vi "Autonomous Independent.vi"() -> ()   [LabVIEW 2017]
doc: "This VI is called when autonomous begins, and will automatically be terminated when autonomous ends. You can carry out timed or sensor driven robot movement independently without needing to return to the caller."
uses:
  <vilib>/Rock Robotics/WPI/ThirdParty/Phoenix-LabVIEW/Motor Controller/Controls/CTRE_Phoenix_MotorControl_FeedbackDevice.ctl
  <vilib>/Rock Robotics/WPI/ThirdParty/Phoenix-LabVIEW/Motor Controller/Controls/CTRE_Phoenix_MotorControl_StatusFrameEnhanced.ctl
  <vilib>/Rock Robotics/WPI/ThirdParty/Phoenix-LabVIEW/Motor Controller/Controls/CTRE_Phoenix_MotorControl_TrajectoryPointTimeDur.ctl
  <vilib>/Utility/file.llb/Read Delimited Spreadsheet (DBL).vi
panel:
  out "Velocity (Sensor Units per 100 ms)":i32
  out "Position (Sensor Units)":i32
  out "Loop Time":u32
  out "Is Last?":bool
  out "Active Point Valid?":bool
  out "Is Underrun?":bool
  out "Has Underrun?":bool
  out "Top Buffer Count":i32
  out "Bottom Buffer Count":i32
  # "Be sure to right-click and choose Data Operations>>Make Current Value default if you want to save the array values with the VI"
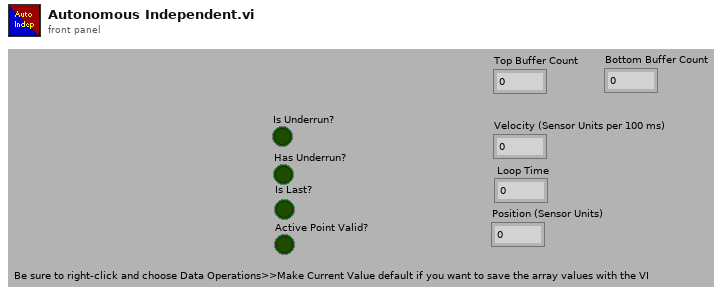
[diagram p1: front panel]
types:
  T1 = typedef "CTRE_Phoenix_MotorControl_StatusFrameEnhanced.ctl" = u16
  T2 = typedef "CTRE_Phoenix_MotorControl_FeedbackDevice.ctl" = i8
  T3 = typedef "WPI_MotorControlDeviceRef.ctl" = cluster{"DeviceStatus":errorcluster, "Type":T4, "PWM":cluster{"PWM Channel":T5, "DeadBand":T6}, "CAN":cluster{"Device Number":u8, "SetOutput VI Ref":variant, "GetOutput VI Ref":variant, "Enable VI Ref":variant, "Disable VI Ref":variant, "Data":variant}, "Invert":bool, "DIO PWM":cluster{"PWM \"Enable\" Channel":T5, "DIOChannel":T7, "PWM Rate":dbl}}
  T4 = typedef "WPI_MotorControlType.ctl" = enum16{"PWM", "CAN", "DIO PWM"}
  T5 = typedef "FPGA_DIOPWMChannel.ctl" = enum8{"PWM 0", "PWM 1", "PWM 2", "PWM 3", "PWM 4", "PWM 5", "PWM 6", "PWM 7", "PWM 8", "PWM 9", "PWM MXP 0", "PWM MXP 1", "PWM MXP 2", "PWM MXP 3", "PWM MXP 4", "PWM MXP 5", "PWM MXP 6", "PWM MXP 7", "PWM MXP 8", "PWM MXP 9", "Invalid"}
  T6 = typedef "WPI_PWMDeadband.ctl" = cluster{"Name":string, "maxPositivePwm":i32, "minPositivePwm":i32, "centerPwm":i32, "maxNegativePwm":i32, "minNegativePwm":i32, "angularRange":u16}
  T7 = typedef "FPGA_DIOChannel.ctl" = enum8{"DIO 0", "DIO 1", "DIO 2", "DIO 3", "DIO 4", "DIO 5", "DIO 6", "DIO 7", "DIO 8", "DIO 9", "DIO MXP 0", "DIO MXP 1", "DIO MXP 2", "DIO MXP 3", "DIO MXP 4", "DIO MXP 5", "DIO MXP 6", "DIO MXP 7", "DIO MXP 8", "DIO MXP 9", "DIO MXP 10", "DIO MXP 11", "DIO MXP 12", "DIO MXP 13", "DIO MXP 14", "DIO MXP 15", "SPI Port CS1", "SPI Port CS2", "SPI Port CS3", "SPI Port MISO", "SPI Port MOSI", "Invalid"}
  T8 = cluster{"Top Buffer Remaining":i32, "Top Buffer Count":i32, "Bottom Buffer Count":i32, "Has Underrun?":bool, "Is Underrun?":bool, "Active Point Valid?":bool, "Is Last?":bool, "Profile Slot Select 0":i32, "Output Enable":i32, "Time Duration (ms)":i32, "Profile Slot Select 1":i32}
  T9 = typedef "CTRE_Phoenix_MotorControl_TrajectoryPointTimeDur.ctl" = i32
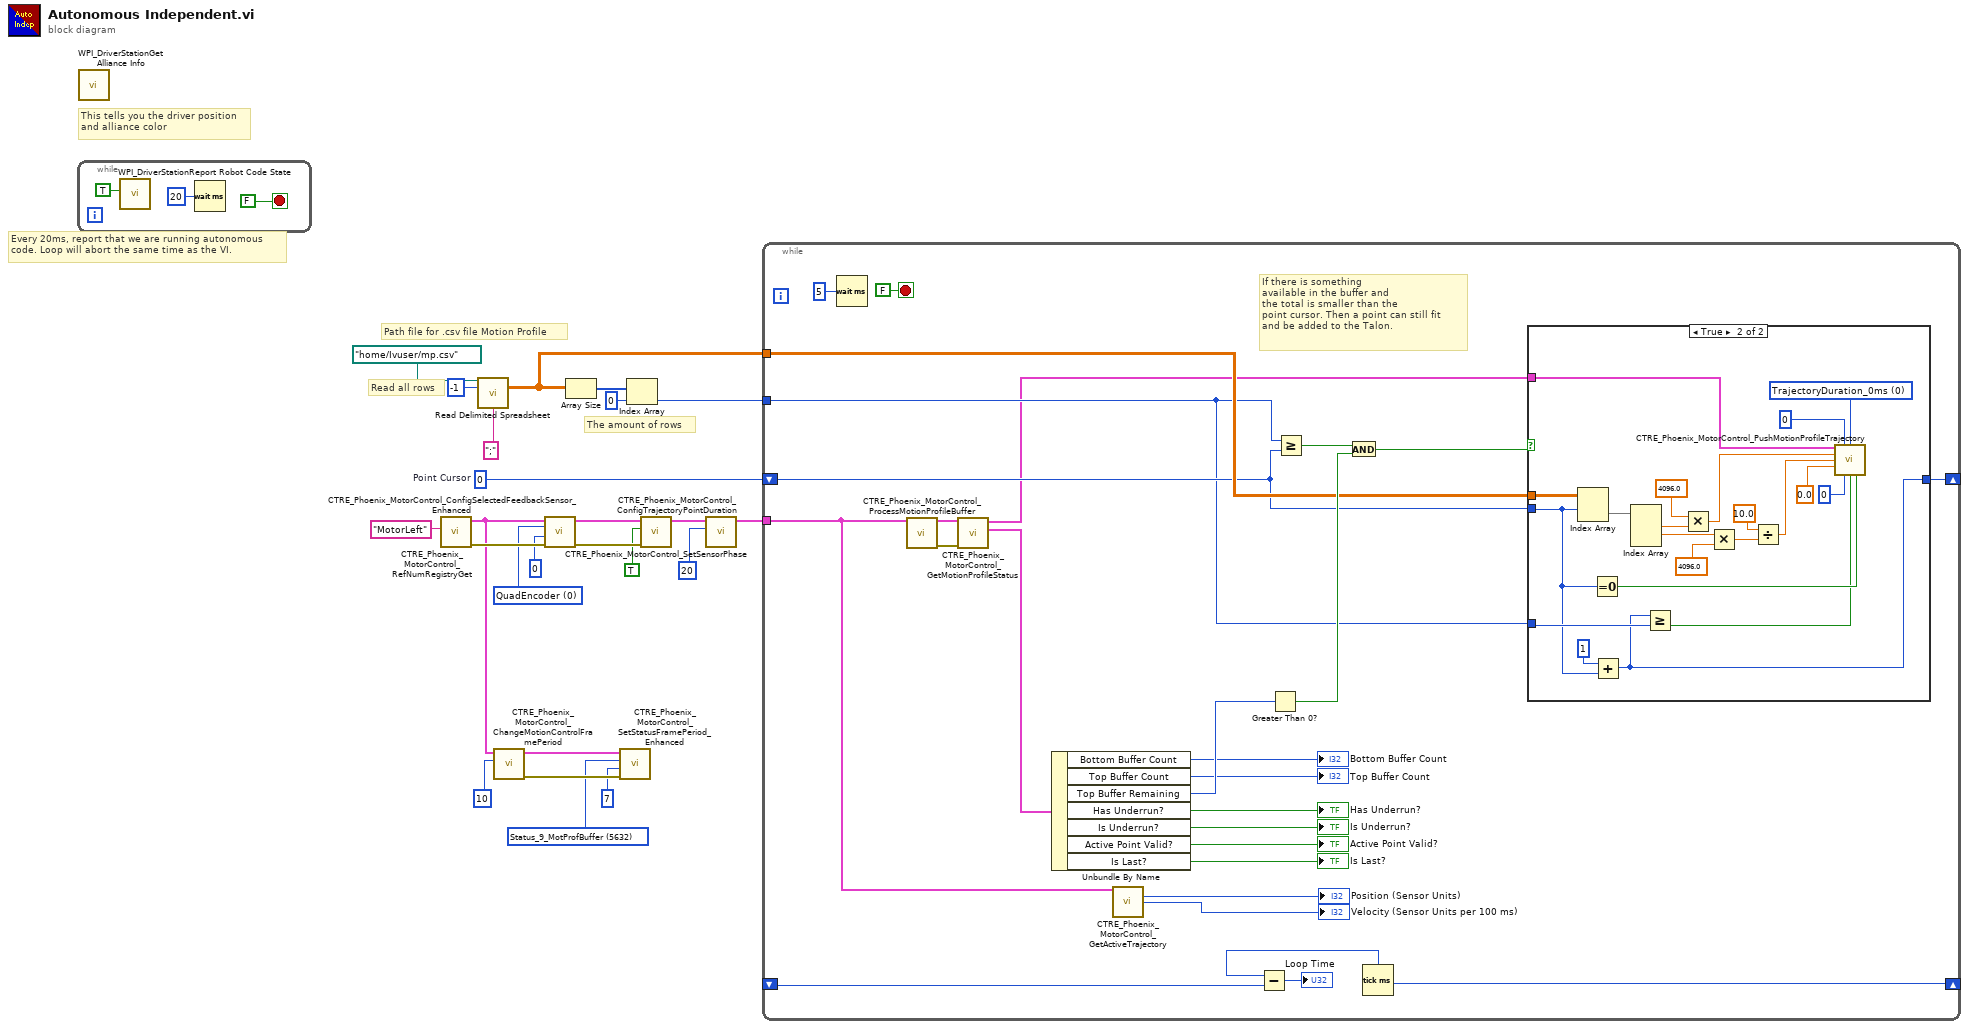
[diagram p0: block diagram]
diagram:
  w1 = 0  # Point Cursor
  w4 = T1 5632 items=["Status_1_General"=5120, "Status_2_Feedback0"=5184, "Status_3_Quadrature"=5248, "Status_4_AinTempVbat"=5312, "Status_6_Misc"=5440, "Status_7_CommStatus"=5504, "Status_8_PulseWidth"=5568, "Status_9_MotProfBuffer"=5632, "Status_10_MotionMagic"=5696, "Status_11_UartGadgeteer"=5760, "Status_12_Feedback1"=5824, "Status_13_Base_PIDF0"=5888, "Status_14_Turn_PIDF1"=5952, "Status_15_FirmwareApiStatus"=6016] ("Status Frame")
  w14 = T2 0 items=["None"=-1, "QuadEncoder"=0, "Analog"=2, "Tachometer"=4, "Pulse Width Encoded Position"=8, "Sensor Sum (S0 + S1)"=9, "Sensor Difference (D0 - D1)"=10, "Remote Source 0"=11, "Remote Source 1"=12, "Software Emulated"=15] ("Feedback Device")
  # "The amount of rows"
  # "Path file for .csv file Motion Profile"
  # "Read all rows"
  # "Every 20ms, report that we are running autonomous\ncode. Loop will abort the same time as the VI."
  # "This tells you the driver position\nand alliance color"
  n1 = while {
    stop <- FALSE stop-if-true
    n2 = call <vilib>:"WPI_DriverStationReport Robot Code State.vi"("Autonomous"=TRUE) -> ()  [unwired: 10 in, 1 out]
    n3 = Wait (ms)(milliseconds to wait=u32 20) -> ()  [unwired: 1 out]
  }
  n4 = call <vilib>:"WPI_DriverStationGet Alliance Info.vi"() -> ()  [unwired: 12 out]
  n5 = call <vilib>:"CTRE_Phoenix_MotorControl_RefNumRegistryGet.vi"("refnum name"="MotorLeft") -> ("error out"=w16:errorcluster, "PhoenixMotorControlDevRef"=w2:T3)  [unwired: 9 in]
  n6 = call-poly <vilib>:"Read Delimited Spreadsheet.vi"("file path (dialog if empty)"=path "/home/Ivuser/mp.csv", "number of rows (all:-1)"=-1, "delimiter (\\t)"=";" ("delimiter (\\t)")) -> ("all rows"=w19:dbl[][])  [unwired: 7 in, 5 out]
  n7 = call <vilib>:"CTRE_Phoenix_MotorControl_ChangeMotionControlFramePeriod.vi"("periodMs"=10, "PhoenixMotorControlDevRef"=w2) -> ("error out"=w5:errorcluster, "PhoenixMotorControlDevRef"=w6:T3)  [unwired: 8 in]
  n8 = call <vilib>:"CTRE_Phoenix_MotorControl_ConfigSelectedFeedbackSensor_Enhanced.vi"("error in (no error)"=w16, "pidLoopIdx"=0, "Feedback Device"=w14, "PhoenixMotorControlDevRef"=w2) -> ("error out"=w12:errorcluster, "PhoenixMotorControlDevRef"=w13:T3)  [unwired: 6 in]
  n9 = Array Size(array=w19) -> (size(s)=w21:i32[])
  n10 = call <vilib>:"CTRE_Phoenix_MotorControl_SetStatusFramePeriod_Enhanced.vi"("error in (no error)"=w5, "periodMs"=7, "Status Frame"=w4, "PhoenixMotorControlDevRef"=w6) -> ()  [unwired: 6 in, 2 out]
  n11 = Index Array(array=w21, index=0) -> (element=w18:i32)
  n12 = call <vilib>:"CTRE_Phoenix_MotorControl_SetSensorPhase.vi"("error in (no error)"=w12, "PhaseSensor"=TRUE, "PhoenixMotorControlDevRef"=w13) -> ("PhoenixMotorControlDevRef"=w10:T3)  [unwired: 7 in, 1 out]
  n13 = call <vilib>:"CTRE_Phoenix_MotorControl_ConfigTrajectoryPointDuration.vi"("durationMs"=20, "PhoenixMotorControlDevRef"=w10) -> ("PhoenixMotorControlDevRef"=w8:T3)  [unwired: 8 in, 1 out]
  n14 = while {
    tunnel: w19 -> [w45]
    tunnel: w18 -> [w43]
    tunnel: w8 -> [w30]
    shift-right: [w40] -> _
    shift-left: w1 -> [w44]
    shift-right: [w32] -> _
    shift-left: _ -> [w33]
    stop <- FALSE stop-if-true
    # "If there is something\navailable in the buffer and\nthe total is smaller than the\npoint cursor. Then a point can still fit\nand be added to the Talon."
    n15 = Wait (ms)(milliseconds to wait=u32 5) -> ()  [unwired: 1 out]
    n16 = call <vilib>:"CTRE_Phoenix_MotorControl_ProcessMotionProfileBuffer.vi"("PhoenixMotorControlDevRef"=w30) -> ("PhoenixMotorControlDevRef"=w50:T3, "error out"=w51:errorcluster)  [unwired: 13 in]
    n17 = call <vilib>:"CTRE_Phoenix_MotorControl_GetMotionProfileStatus.vi"("error in"=w51, "PhoenixMotorControlDevRef"=w50) -> ("Motion Profile Status"=w49:T8, "PhoenixMotorControlDevRef"=w42:T3)  [unwired: 7 in, 1 out]
    n18 = Unbundle By Name(w49) -> ("Bottom Buffer Count"=→"Bottom Buffer Count":i32, "Top Buffer Count"=→"Top Buffer Count":i32, "Top Buffer Remaining"=w41:i32, "Has Underrun?"=→"Has Underrun?":bool, "Is Underrun?"=→"Is Underrun?":bool, "Active Point Valid?"=→"Active Point Valid?":bool, "Is Last?"=→"Is Last?":bool)
    n19 = call <vilib>:"CTRE_Phoenix_MotorControl_GetActiveTrajectory.vi"("PhoenixMotorControlDevRef"=w30) -> ("Position (Sensor Units)"=→"Position (Sensor Units)":i32, "Velocity (Sensor Units per 100 ms)"=→"Velocity (Sensor Units per 100 ms)":i32)  [unwired: 10 in, 3 out]
    n20 = Greater Than 0?(x=w41) -> (x > 0?=w47:bool)
    n21 = Greater Or Equal?(x=w43, y=w44) -> (x >= y?=w48:bool)
    n22 = And(x=w48, y=w47) -> (x .and. y?=w46:bool)
    n23 = Tick Count (ms)() -> (millisecond timer value=w32:u32)
    n24 = Subtract(x=w32, y=w33) -> (x-y=→"Loop Time":u32)
    n25 = case shown="True" w46 {
      tunnel: w45 -> [_ w75]
      tunnel: w44 -> [w54 w62]
      tunnel: w43 -> [_ w63]
      tunnel: w42 -> [_ w60]
      tunnel: [w54 w59] -> w40
      frame False {
      }
      frame True {
        w55 = T9 0 items=["TrajectoryDuration_0ms"=0, "TrajectoryDuration_5ms"=5, "TrajectoryDuration_10ms"=10, "TrajectoryDuration_20ms"=20, "TrajectoryDuration_30ms"=30, "TrajectoryDuration_40ms"=40, "TrajectoryDuration_50ms"=50, "TrajectoryDuration_100ms"=100] ("durationMs")
        n26 = Index Array(array=w75, index (row)=w62) -> (element=w74:dbl[])  [unwired: 1 in]
        n27 = Equal To 0?(x=w62) -> (x = 0?=w65:bool)
        n28 = Add(x=1, y=w62) -> (x+y=w59:i32)
        n29 = Index Array(array=w74) -> (element #1=w73:dbl, element #2=w71:dbl)  [unwired: 3 in, 1 out]
        n30 = Greater Or Equal?(x=w59, y=w63) -> (x >= y?=w61:bool)
        n31 = Multiply(x=4096.0 ("element"), y=w73) -> (x*y=w67:dbl)
        n32 = Multiply(x=w71, y=4096.0) -> (x*y=w69:dbl)
        n33 = Divide(x=10.0, y=w69) -> (x/y=w66:dbl)
        n34 = call <vilib>:"CTRE_Phoenix_MotorControl_PushMotionProfileTrajectory.vi"("PhoenixMotorControlDevRef"=w60, "profileSlotSelect1"=0, "durationMs"=w55, "position"=w67, "velocity"=w66, "auxiliaryPos"=0.0, "profileSlotSelect0"=0, "isLastPoint?"=w61, "Zero Position?"=w65) -> ()  [unwired: 5 in, 2 out]
      }
    }
  }
